vi "Update_Ch_Names.vi"(1 "Ch Name in":string[](array[string])) -> (0 "Ch Name Out":string[](array[string]))   [LabVIEW 2022 SP3]
uses:
  Globals/Meas_global.vi
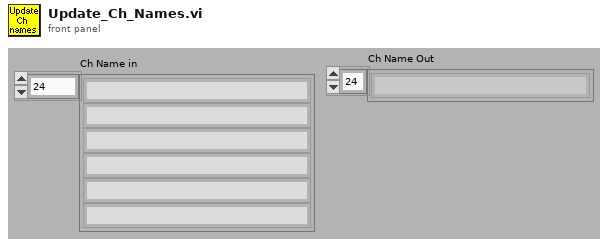
[diagram p1: front panel]
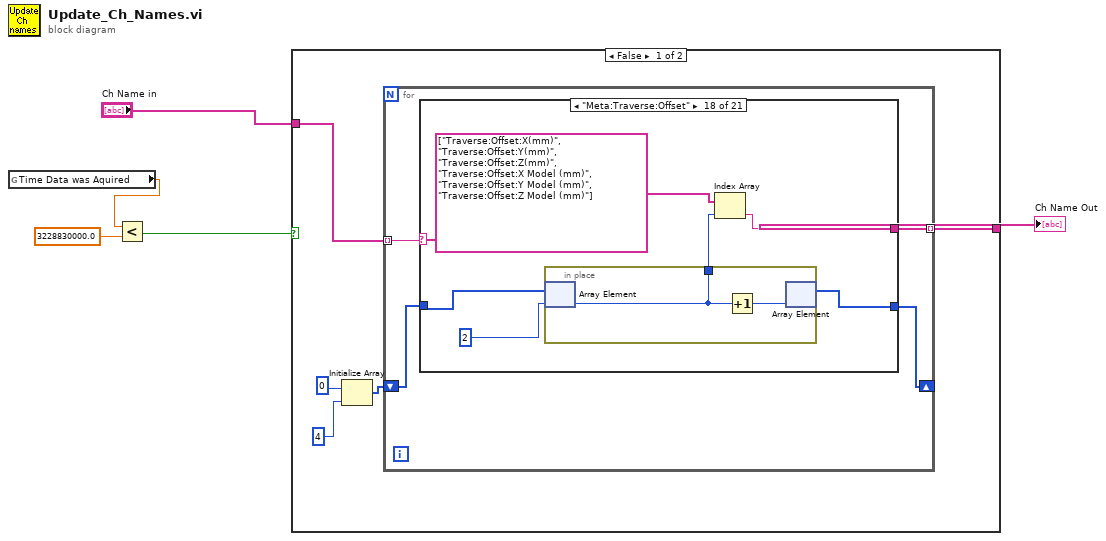
[diagram p0: block diagram]
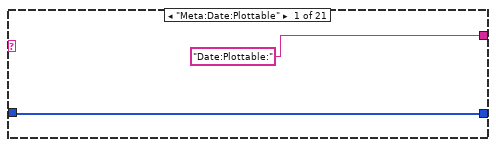
[diagram p2: hidden frame]
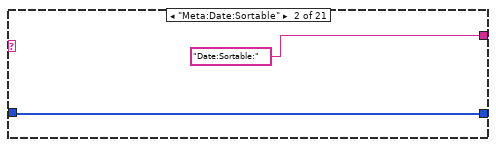
[diagram p3: hidden frame]
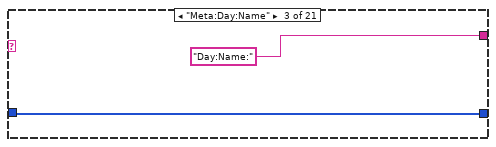
[diagram p4: hidden frame]
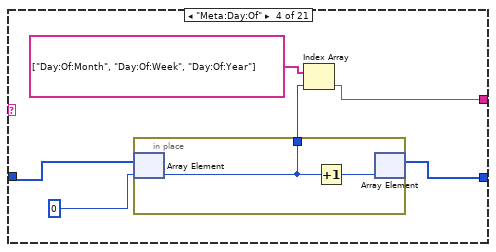
[diagram p5: hidden frame]
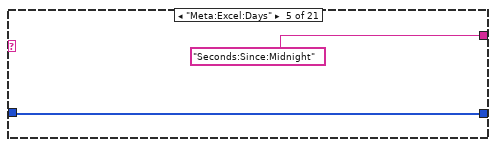
[diagram p6: hidden frame]
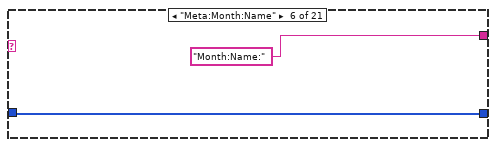
[diagram p7: hidden frame]
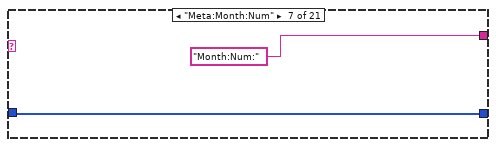
[diagram p8: hidden frame]
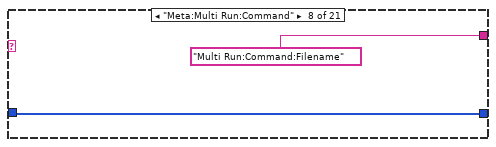
[diagram p9: hidden frame]
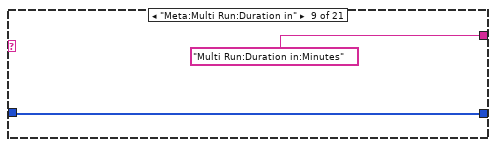
[diagram p10: hidden frame]
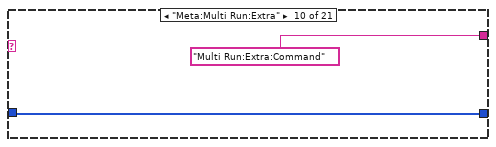
[diagram p11: hidden frame]
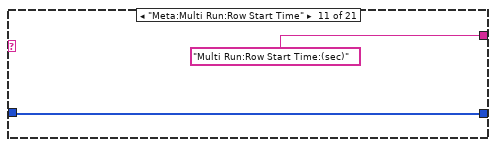
[diagram p12: hidden frame]
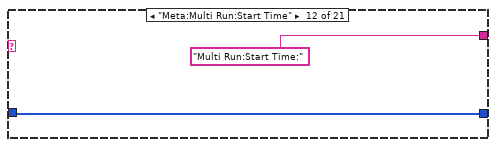
[diagram p13: hidden frame]
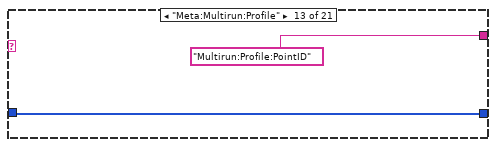
[diagram p14: hidden frame]
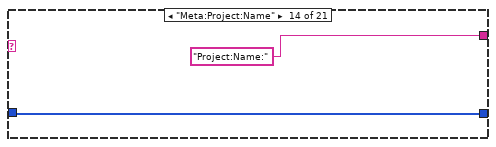
[diagram p15: hidden frame]
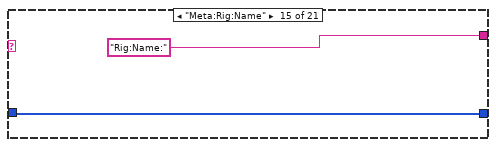
[diagram p16: hidden frame]
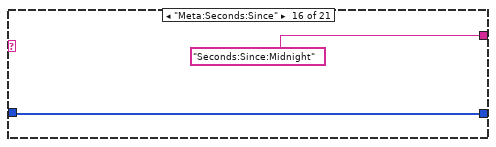
[diagram p17: hidden frame]
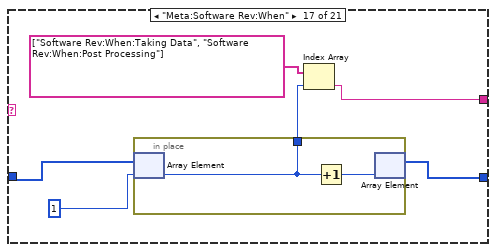
[diagram p18: hidden frame]
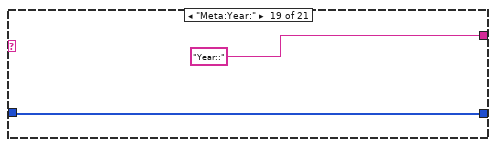
[diagram p19: hidden frame]
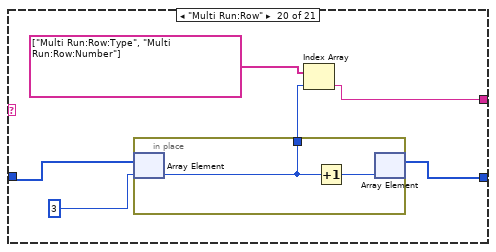
[diagram p20: hidden frame]
diagram:
  n1 = global read "Meas_global.vi" "Time Data was Aquired"() -> (w3:dbl)
  n2 = Less?(x=w3, y=3228830000.0) -> (x < y?=w1:bool)
  n3 = case shown="False" w1 {
    tunnel: "Ch Name in" -> [w10 w82]
    tunnel: [w9 w81] -> w4
    frame False {
      n4 = Initialize Array(0, 4 ("dimension size")) -> (w6:i32[])
      n5 = for {
        tunnel: w10 -> [w14] mode=indexing
        tunnel: [w13] -> w9 mode=indexing
        shift-right: [w12] -> _
        shift-left: w6 -> [w11]
        n6 = case shown="\"Meta:Traverse:Offset\"" w14 {
          selector: w14 -> [_ _ _ _ _ _ _ _ _ _ _ _ _ _ _ _ _ _ _ _ w80]
          tunnel: ["Date:Plottable:" "Date:Sortable:" "Day:Name:" w21 "Seconds:Since:Midnight" "Month:Name:" "Month:Num:" "Multi Run:Command:Filename" "Multi Run:Duration in:Minutes" "Multi Run:Extra:Command" "Multi Run:Row Start Time:(sec)" "Multi Run:Start Time:" "Multirun:Profile:PointID" "Project:Name:" "Rig:Name:" "Seconds:Since:Midnight" w53 w61 "Year::" w71 w80] -> w13
          tunnel: [w15 w17 w19 w24 w29 w31 w33 w35 w37 w39 w41 w43 w45 w47 w49 w51 w56 w64 w69 w74 w79] -> w12
          tunnel: w11 -> [w15 w17 w19 w26 w29 w31 w33 w35 w37 w39 w41 w43 w45 w47 w49 w51 w58 w66 w69 w76 w79]
          frame "Meta:Date:Plottable" {
          }
          frame "Meta:Date:Sortable" {
          }
          frame "Meta:Day:Name" {
          }
          frame "Meta:Day:Of" {
            n7 = in-place {
              in-place-border: [w28] -> w22
              n8 = in-place-array #1(w26, 0) -> (w28:i32)
              n9 = Increment(x=w28) -> (x+1=w27:i32)
              n10 = in-place-array #1(w27) -> (w24:i32[])  [unwired: 1 out]
            }
            n11 = Index Array(array=string[] ["Day:Of:Month", "Day:Of:Week", "Day:Of:Year"], index=w22) -> (element=w21:string)
          }
          frame "Meta:Excel:Days" {
          }
          frame "Meta:Month:Name" {
          }
          frame "Meta:Month:Num" {
          }
          frame "Meta:Multi Run:Command" {
          }
          frame "Meta:Multi Run:Duration in" {
          }
          frame "Meta:Multi Run:Extra" {
          }
          frame "Meta:Multi Run:Row Start Time" {
          }
          frame "Meta:Multi Run:Start Time" {
          }
          frame "Meta:Multirun:Profile" {
          }
          frame "Meta:Project:Name" {
          }
          frame "Meta:Rig:Name" {
          }
          frame "Meta:Seconds:Since" {
          }
          frame "Meta:Software Rev:When" {
            n12 = in-place {
              in-place-border: [w60] -> w54
              n13 = in-place-array #2(w58, 1) -> (w60:i32)
              n14 = Increment(x=w60) -> (x+1=w59:i32)
              n15 = in-place-array #2(w59) -> (w56:i32[])  [unwired: 1 out]
            }
            n16 = Index Array(array=string[] ["Software Rev:When:Taking Data", "Software Rev:When:Post Processing"], index=w54) -> (element=w53:string)
          }
          frame "Meta:Traverse:Offset" {
            n17 = in-place {
              in-place-border: [w68] -> w62
              n18 = in-place-array #3(w66, 2) -> (w68:i32)
              n19 = Increment(x=w68) -> (x+1=w67:i32)
              n20 = in-place-array #3(w67) -> (w64:i32[])  [unwired: 1 out]
            }
            n21 = Index Array(array=string[] ["Traverse:Offset:X(mm)", "Traverse:Offset:Y(mm)", "Traverse:Offset:Z(mm)", "Traverse:Offset:X Model (mm)", "Traverse:Offset:Y Model (mm)", "Traverse:Offset:Z Model (mm)"], index=w62) -> (element=w61:string)
          }
          frame "Meta:Year:" {
          }
          frame "Multi Run:Row" {
            n22 = in-place {
              in-place-border: [w78] -> w72
              n23 = in-place-array #4(w76, 3) -> (w78:i32)
              n24 = Increment(x=w78) -> (x+1=w77:i32)
              n25 = in-place-array #4(w77) -> (w74:i32[])  [unwired: 1 out]
            }
            n26 = Index Array(array=string[] ["Multi Run:Row:Type", "Multi Run:Row:Number"], index=w72) -> (element=w71:string)
          }
          frame Default {
          }
        }
      }
    }
    frame True {
      n27 = for {
        tunnel: w82 -> [w88] mode=indexing
        tunnel: [w84] -> w81 mode=indexing
        n28 = call "Fast_string_Replace.vi"("Replace match with:"="EnFlo_Tunnel:" ("regular expression"), "Input String"=w88, "matchThis"="EnFlo Tun:" ("regular expression")) -> ("Output String"=w83:string)  [unwired: 1 in, 1 out]
        n29 = call "Fast_string_Replace.vi"("Replace match with:"="_Tunnel" ("regular expression"), "Input String"=w83, "matchThis"=" Tunnel" ("regular expression")) -> ("Output String"=w84:string)  [unwired: 1 in, 1 out]
      }
    }
  }
  "Ch Name Out" <- w4
